vi "CMN_Str2Arr.vi"(6 "trim":bool=TRUE, 7 "strip quotation marks":bool, 9 "separator":string=",", 10 "string in":string) -> (2 "Array out":string[](array[string]))   [LabVIEW 2016]
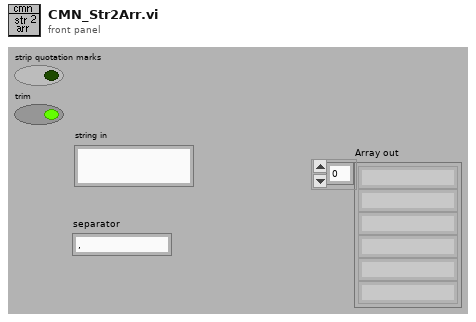
[diagram p1: front panel]
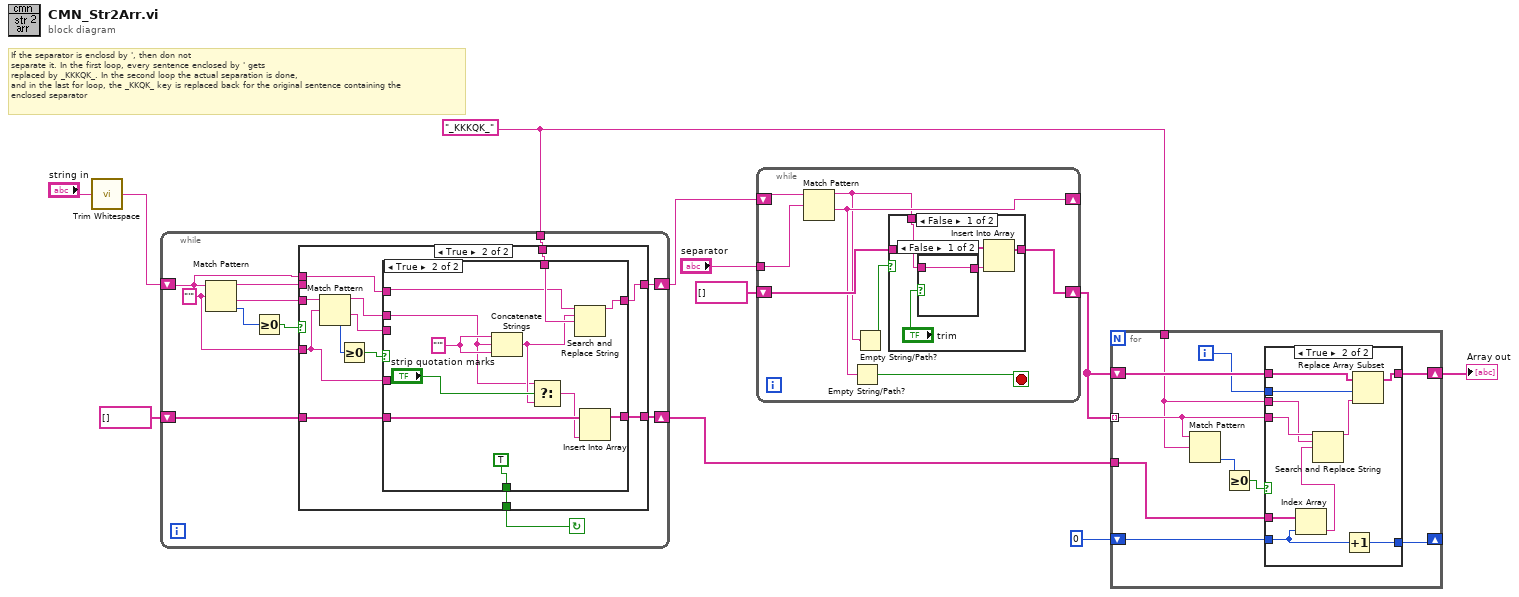
[diagram p0: block diagram]
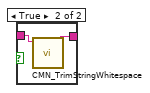
[diagram p3: hidden frame]
diagram:
  w4 = "_KKKQK_" ("replace string (\"\")")
  # "If the separator is enclosd by ', then don not\nseparate it. In the first loop, every sentence enclosed by ' gets\nreplaced by _KKKQK_. In the second loop the actual separation is done,\nand in the last for loop, the _KKQK_ key is replaced back for the original sentence containing the \nenclosed separator"
  n1 = call <vilib>:"Trim Whitespace.vi"("string"="string in") -> ("trimmed string"=w10:string)  [unwired: 1 in]
  n2 = while {
    shift-right: [w17] -> w9
    shift-left: w10 -> [w18]
    tunnel: w4 -> [w14]
    shift-right: [w13] -> w5
    shift-left: string[] [] -> [w12]
    stop <- w16 continue-if-true
    w19 = "'" ("regular expression")
    n3 = Match Pattern(string=w18, regular expression=w19) -> (before substring=w15:string, after substring=w20:string, offset past match=w22:i32)  [unwired: 2 out]
    n4 = Greater Or Equal To 0?(x=w22) -> (x >= 0?=w21:bool)
    n5 = case shown="True" w21 {
      selector: w21 -> [w24 _]
      tunnel: w20 -> [_ w36]
      tunnel: w19 -> [_ w29]
      tunnel: w18 -> [w25 w34]
      tunnel: [w25 w33] -> w17
      tunnel: [w24 w32] -> w16
      tunnel: w15 -> [_ _]
      tunnel: w14 -> [_ w28]
      tunnel: [w23 w27] -> w13
      tunnel: w12 -> [w23 w26]
      frame False {
      }
      frame True {
        n6 = Match Pattern(string=w36, regular expression=w29) -> (before substring=w31:string, after substring=w30:string, offset past match=w37:i32)  [unwired: 2 out]
        n7 = Greater Or Equal To 0?(x=w37) -> (x >= 0?=w35:bool)
        n8 = case shown="True" w35 {
          selector: w35 -> [w39 _]
          tunnel: w34 -> [w40 w47]
          tunnel: [w40 w46] -> w33
          tunnel: [w39 TRUE] -> w32
          tunnel: w31 -> [_ w42]
          tunnel: w30 -> [_ _]
          tunnel: w29 -> [_ _]
          tunnel: w28 -> [_ w50]
          tunnel: [w38 w49] -> w27
          tunnel: w26 -> [w38 w48]
          frame False {
          }
          frame True {
            w45 = "'" ("string")
            n9 = Concatenate Strings(w45, w42, w45) -> (w43:string)
            n10 = Select(t=w42, s="strip quotation marks", f=w43) -> (s? t:f=w41:string)
            n11 = Search and Replace String(input string=w47, search string=w43, replace string=w50) -> (result string=w46:string)  [unwired: 1 in, 7 out]
            n12 = Insert Into Array(array=w48, new element=w41) -> (w49:string[])  [unwired: 1 in]
          }
        }
      }
    }
  }
  n13 = while {
    shift-right: [w55] -> _
    shift-left: w9 -> [w59]
    tunnel: "separator" -> [w58]
    shift-right: [w57] -> w3
    shift-left: string[] [] -> [w56]
    stop <- w54 stop-if-true
    n14 = Match Pattern(string=w59, regular expression=w58) -> (before substring=w53:string, after substring=w55:string)  [unwired: 3 out]
    n15 = Empty String/Path?(string/path=w55) -> (empty?=w54:bool)
    n16 = Empty String/Path?(string/path=w53) -> (empty?=w52:bool)
    n17 = case shown="False" w52 {
      tunnel: w53 -> [w62 _]
      tunnel: [w64 w68] -> w57
      tunnel: w56 -> [w63 w68]
      frame False {
        n18 = case shown="False" "trim" {
          tunnel: w62 -> [w65 w67]
          tunnel: [w65 w66] -> w61
          frame False {
          }
          frame True {
            n19 = call "CMN_TrimStringWhitespace.vi"("string"=w67) -> ("trimmed string"=w66:string)  [unwired: 1 in, 8 out]
          }
        }
        n20 = Insert Into Array(array=w63, new element=w61) -> (w64:string[])  [unwired: 1 in]
      }
      frame True {
      }
    }
  }
  n21 = for {
    tunnel: w3 -> [w75] mode=indexing
    tunnel: w5 -> [w74]
    tunnel: w4 -> [w71]
    shift-right: [w69] -> w1
    shift-left: w3 -> [w76]
    shift-right: [w72] -> _
    shift-left: 0 -> [w73]
    i -> [w70]
    n22 = Match Pattern(string=w75, regular expression=w71) -> (offset past match=w78:i32)  [unwired: 4 out]
    n23 = Greater Or Equal To 0?(x=w78) -> (x >= 0?=w77:bool)
    n24 = case shown="True" w77 {
      tunnel: w76 -> [w80 w84]
      tunnel: w75 -> [_ w90]
      tunnel: w74 -> [_ w89]
      tunnel: w73 -> [w79 w88]
      tunnel: [w79 w87] -> w72
      tunnel: w71 -> [_ w86]
      tunnel: w70 -> [_ w83]
      tunnel: [w80 w81] -> w69
      frame False {
      }
      frame True {
        n25 = Index Array(array=w89, index=w88) -> (element=w85:string)
        n26 = Search and Replace String(input string=w90, search string=w86, replace string=w85) -> (result string=w82:string)  [unwired: 1 in, 7 out]
        n27 = Increment(x=w88) -> (x+1=w87:i32)
        n28 = Replace Array Subset(array=w84, new element=w82, index=w83) -> (w81:string[])
      }
    }
  }
  "Array out" <- w1
